vi "MICSD Send MICS Data.vi"(8 "error in (no error)":errorcluster, 9 "BlockSize":u8=15, 10 "Send Data":u8[](array[numeric]) format="%02x", 11 "VISA Resource Name":refnum<visa-resource-name>) -> (0 "error out":errorcluster, 3 "dup VISA Resource Name":refnum<visa-resource-name>)   [LabVIEW 2020]
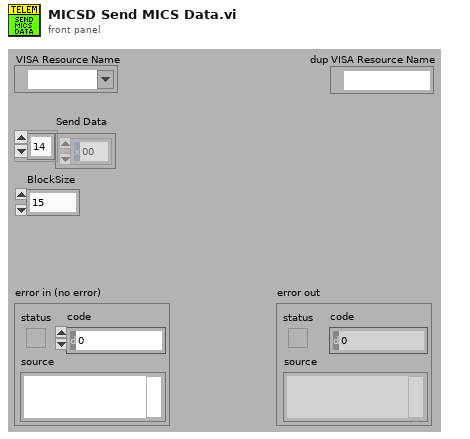
[diagram p1: front panel]
types:
  T1 = cluster{"Command Token":u8, "Length":u16, "Pack Data":u8[]}
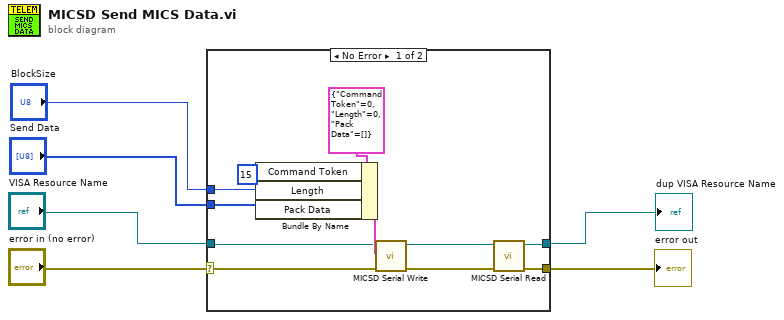
[diagram p0: block diagram]
diagram:
  n1 = case shown="No Error" "error in (no error)" {
    selector: "error in (no error)" -> [w13 w19]
    tunnel: [w8 w19] -> w3
    tunnel: "VISA Resource Name" -> [w12 w18]
    tunnel: [w11 w18] -> w4
    tunnel: "Send Data" -> [w10 _]
    tunnel: "BlockSize" -> [w9 _]
    frame No Error {
      n2 = Bundle By Name(cluster=T1 {"Command Token"=0, "Length"=0, "Pack Data"=[]} ("Write Data"), "Command Token"=u8 15, "Length"=w9, "Pack Data"=w10) -> (w17:T1)
      n3 = call "MICSD Serial Write.vi"("error in (no error)"=w13, "Write Data"=w17, "VISA Resource Name"=w12) -> ("error out"=w7:errorcluster, "DUP Visa Resource Name"=w15:refnum<visa-resource-name>)  [unwired: 7 in]
      n4 = call "MICSD Serial Read.vi"("error in (no error)"=w7, "VISA Resource Name"=w15) -> ("error out"=w8:errorcluster, "DUP Visa Resource Name"=w11:refnum<visa-resource-name>)  [unwired: 7 in, 1 out]
    }
    frame Error {
    }
  }
  "dup VISA Resource Name" <- w4
  "error out" <- w3
